vi "ingest.dataflash_add_file_tag.vi"(8 "error in":errorcluster, 11 "DataflashIngestStaging in":refnum<class "DataflashIngestStaging.lvclass">) -> (0 "error out":errorcluster, 3 "DataflashIngestStaging out":refnum<class "DataflashIngestStaging.lvclass">)   [LabVIEW 2020, in "DataflashIngestStaging.lvclass"]
doc: "Applies a fixed tag and value to every record ingested from the DataFlash file."
uses:
  DataflashIngestStaging.lvclass
  DataflashIngestStaging.lvclass/DataflashIngestStaging.ctl
  client.lvlib
panel:
  in  "tag":string
  in  "value":string
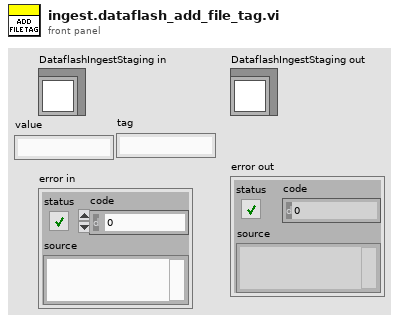
[diagram p1: front panel]
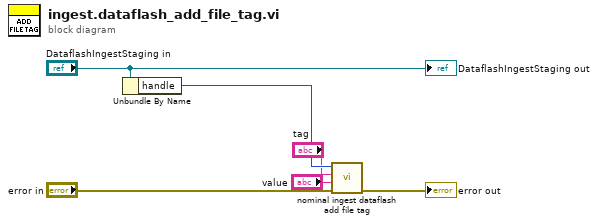
[diagram p0: block diagram]
diagram:
  n1 = Unbundle By Name("DataflashIngestStaging in") -> ("handle"=w4:i32)
  n2 = call "nominal ingest dataflash add file tag.vi"("error in (no error)"="error in", "value"="value", "tag"="tag", "staging"=w4) -> ("error out"=→"error out":errorcluster)  [unwired: 6 in, 1 out]
  "DataflashIngestStaging out" <- "DataflashIngestStaging in"
